vi "ConfigureLowRateAnalysis.vi"(8 "error in (no error)":errorcluster) -> (0 "error out":errorcluster, 2 "register trends":T1[](array[typedef]), 3 "analysis config":T3, 5 "all config found?":bool)   [LabVIEW 2017, in "McsaAnalysisLowRate.lvlib"]
uses:
  <vilib>/addons/InsightCM/Devices/Shared/Mcsa/McsaAnalysisLowRate/McsaAnalysisLowRate.lvlib
  <vilib>/addons/InsightCM/Utilities/GlobalConfiguration/GlobalConfiguration.lvlib
  <vilib>/addons/InsightCM/Utilities/DeviceModelHelpers/DeviceModelHelpers.lvlib
  <vilib>/addons/InsightCM/Utilities/Analysis/Shared/AnalysisHelper.lvlib
  <vilib>/addons/InsightCM/Devices/Shared/Mcsa/McsaVirtualChannel/McsaVirtualChannel.lvlib
  <vilib>/addons/InsightCM/Utilities/Analysis/MCSA/McsaAnalysisFunctions.lvlib
  <vilib>/addons/InsightCM/Utilities/Analysis/Shared/controls/AmplitudeScale.ctl
  <vilib>/addons/InsightCM/Utilities/Analysis/Shared/controls/Feature.ctl
  <vilib>/addons/InsightCM/Utilities/Analysis/MCSA/controls/McsaChannelPhasor.ctl
  <vilib>/addons/InsightCM/Devices/Shared/Mcsa/McsaAnalysisLowRate/controls/Group.ctl
  <vilib>/addons/InsightCM/Utilities/Analysis/MCSA/controls/WorkingCurrent.ctl
  <vilib>/addons/InsightCM/Devices/Shared/Mcsa/McsaAnalysisLowRate/controls/Config.ctl
  <vilib>/addons/InsightCM/Utilities/Analysis/MCSA/controls/McsaChannel.ctl
  <vilib>/addons/InsightCM/MessageBus/Base/controls/KeyValuePair.ctl
  <vilib>/addons/InsightCM/Utilities/Analysis/MCSA/controls/McsaMotor.ctl
  <vilib>/addons/InsightCM/Utilities/Analysis/MCSA/controls/TorqueLoadEfficiency.ctl
  <vilib>/addons/Electrical Power/Basic/Measurement/subVIs/basic_Power Value.ctl
  <vilib>/addons/Electrical Power/Basic/NI_EP_Basic.lvlib
  <vilib>/addons/InsightCM/Utilities/Analysis/MCSA/controls/MotorCalculationCache.ctl
  <vilib>/addons/InsightCM/Devices/Shared/Common/DataEventCreator/controls/Registry_Trend.ctl
  <vilib>/addons/InsightCM/Devices/Shared/Common/DataEventCreator/DataEventCreator.lvlib
  <vilib>/addons/InsightCM/Devices/Shared/Common/DataEventCreator/controls/RegisterTrendPoints.ctl
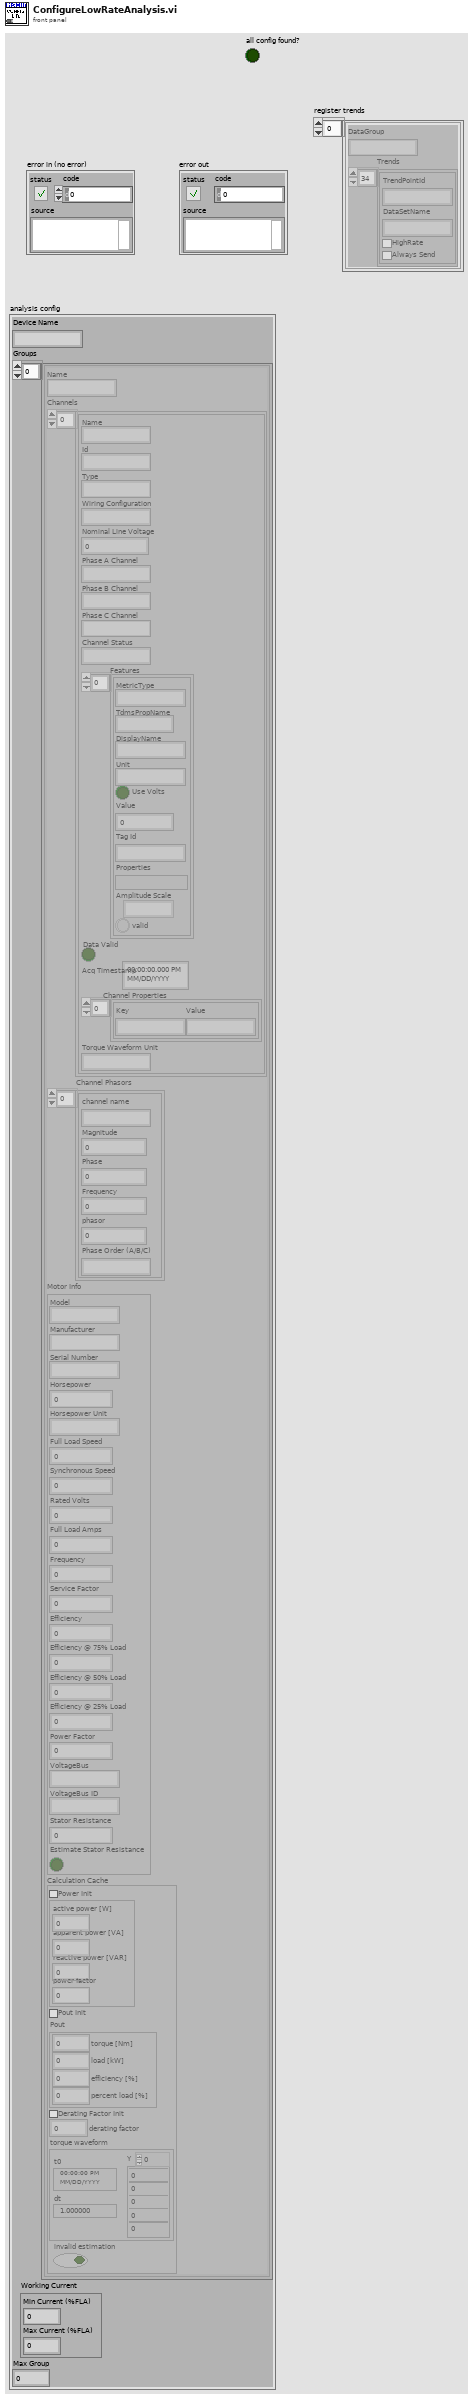
[diagram p1: front panel]
types:
  T1 = typedef "DataEventCreator.lvlib/RegisterTrendPoints.ctl" = cluster{"DataGroup":string, "Trends":T2[]}
  T2 = typedef "DataEventCreator.lvlib/Registry_Trend.ctl" = cluster{"TrendPointId":string, "DataSetName":string, "HighRate":bool, "Always Send":bool}
  T3 = typedef "McsaAnalysisLowRate.lvlib/Config.ctl" = cluster{"Device Name":string, "Groups":T4[], "Working Current":T14, "Max Group":i32}
  T4 = typedef "McsaAnalysisLowRate.lvlib/Group.ctl" = cluster{"Name":string, "Channels":T5[], "Channel Phasors":T9[], "Motor Info":T10, "Calculation Cache":T11}
  T5 = typedef "McsaAnalysisFunctions.lvlib/McsaChannel.ctl" = cluster{"Name":string, "Id":string, "Type":string, "Wiring Configuration":string, "Nominal Line Voltage":dbl, "Phase A Channel":string, "Phase B Channel":string, "Phase C Channel":string, "Channel Status":string, "Features":T6[], "Data Valid":bool, "Acq Timestamp":timestamp, "Channel Properties":T8[], "Torque Waveform Unit":string}
  T6 = typedef "AnalysisHelper.lvlib/Feature.ctl" = cluster{"MetricType":string, "TdmsPropName":string, "DisplayName":string, "Unit":string, "Use Volts":bool, "Value":dbl, "Tag Id":string, "Properties":variant, "Amplitude Scale":T7, "valid":bool}
  T7 = typedef "AnalysisHelper.lvlib/AmplitudeScale.ctl" = enum16{"rms", "peak", "pk-pk"}
  T8 = typedef "KeyValuePair.ctl" = cluster{"Key":string, "Value":string}
  T9 = typedef "McsaAnalysisFunctions.lvlib/McsaChannelPhasor.ctl" = cluster{"channel name":string, "Magnitude":dbl, "Phase":dbl, "Frequency":dbl, "phasor":cdb, "Phase Order (A/B/C)":string}
  T10 = typedef "McsaAnalysisFunctions.lvlib/McsaMotor.ctl" = cluster{"Model":string, "Manufacturer":string, "Serial Number":string, "Horsepower":dbl, "Horsepower Unit":string, "Full Load Speed":dbl, "Synchronous Speed":dbl, "Rated Volts":dbl, "Full Load Amps":dbl, "Frequency":dbl, "Service Factor":dbl, "Efficiency":dbl, "Efficiency @ 75% Load":dbl, "Efficiency @ 50% Load":dbl, "Efficiency @ 25% Load":dbl, "Power Factor":dbl, "VoltageBus":string, "VoltageBus ID":string, "Stator Resistance":dbl, "Estimate Stator Resistance":bool}
  T11 = typedef "McsaAnalysisFunctions.lvlib/MotorCalculationCache.ctl" = cluster{"Power Init":bool, "power value":T12, "Pout Init":bool, "Pout":T13, "Derating Factor Init":bool, "derating factor":sgl, "torque waveform":waveform(dbl), "invalid estimation":bool}
  T12 = typedef "NI_EP_Basic.lvlib/basic_Power Value.ctl" = cluster{"active power [W]":dbl, "apparent power [VA]":dbl, "reactive power [VAR]":dbl, "power factor":dbl}
  T13 = typedef "McsaAnalysisFunctions.lvlib/TorqueLoadEfficiency.ctl" = cluster{"torque [Nm]":dbl, "load [kW]":dbl, "efficiency [%]":dbl, "percent load [%]":dbl}
  T14 = typedef "McsaAnalysisFunctions.lvlib/WorkingCurrent.ctl" = cluster{"Min Current (%FLA)":dbl, "Max Current (%FLA)":dbl}
  T15 = typedef "R2_DeviceModel.ctl" = cluster{"Device":T16, "Channels":T23[], "Tags":T25[]}
  T16 = typedef "R2_Device.ctl" = cluster{"Id":string, "Name":string, "DeviceType":string, "HardwareName":string, "IpAddress":string, "HardwareInfo":T8[], "ApplicationType":string, "ApplicationVersion":string, "EquipmentIds":string[], "ConfigurationVersion":string, "State":T17, "Properties":T8[], "DataGroups":T18[], "BurstModeTrigger":T22}
  T17 = typedef "DeviceState.ctl" = cluster{"Disabled":bool}
  T18 = typedef "R2_DataGroup.ctl" = cluster{"Name":string, "OperatingStates":T19[], "Properties":T8[], "EquipmentIds":string[], "AssetNodeId":string}
  T19 = typedef "OperatingState.ctl" = cluster{"Name":string, "Properties":T8[], "Triggers":T20[]}
  T20 = typedef "Trigger.ctl" = cluster{"Type":string, "Expression":string, "Conditions":T21[]}
  T21 = typedef "Condition.ctl" = cluster{"Source":string, "Type":string, "Operator":string, "CompareTo":string, "DwellSeconds":dbl}
  T22 = typedef "BurstModeTrigger.ctl" = cluster{"Trigger":T20, "SampleRate":string, "AcquisitionLength":string}
  T23 = typedef "R2_Channel.ctl" = cluster{"Id":string, "DeviceId":string, "Name":string, "ChannelType":string, "HardwareKey":string, "HardwareChannel":string, "DataGroup":string, "Keywords":string[], "EquipmentIds":string[], "Properties":T8[], "Metrics":T24[], "AssetNodeId":string, "MeasType":string, "AssetName":string}
  T24 = typedef "Metric.ctl" = cluster{"Id":string, "Name":string, "Unit":string, "Properties":T8[], "MetricDefinitionInstanceId":string}
  T25 = typedef "Tag.ctl" = cluster{"Id":string, "Path":string, "Name":string, "Datatype":string, "Props":T8[], "Keywords":string[]}
  T26 = typedef "SectionKeyValues.ctl" = cluster{"Section":string, "KeyValues":T8[]}
  T27 = typedef "MetricDefinitionInstance.ctl" = cluster{"Id":string, "MetricType":string, "Name":string, "Properties":T8[], "HighRate":bool}
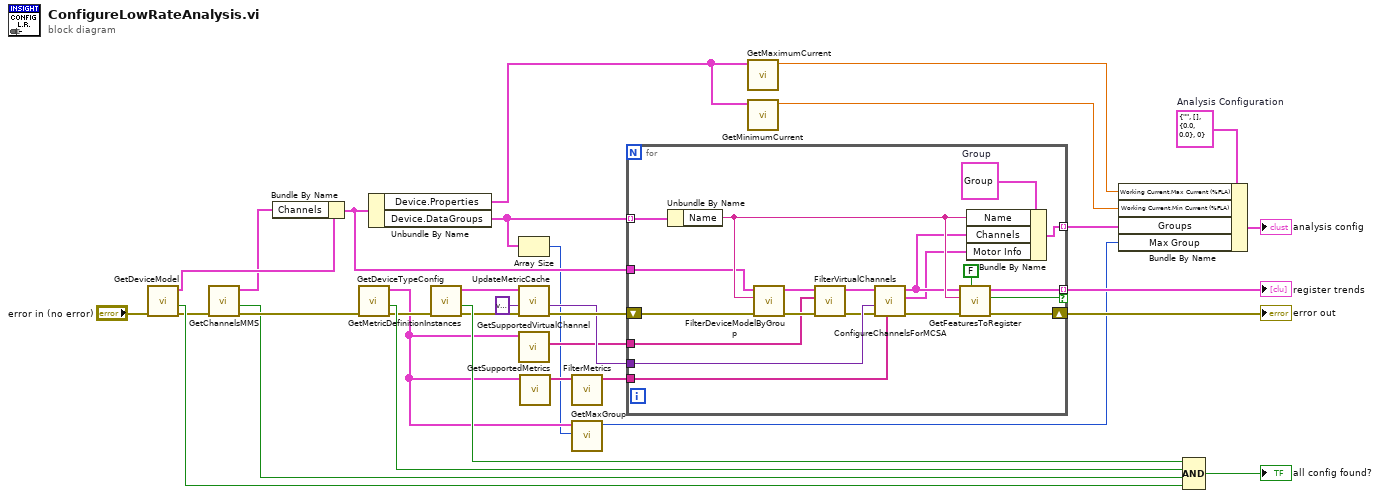
[diagram p0: block diagram]
diagram:
  w10 = T3 {"Device Name"="", "Groups"=[], "Working Current"={"Min Current (%FLA)"=0.0, "Max Current (%FLA)"=0.0}, "Max Group"=0}  # Analysis Configuration
  n1 = call <vilib>:"GetDeviceModel.vi"("error in (no error)"="error in (no error)") -> ("error out"=w13:errorcluster, "found"=w28:bool, "device model"=w15:T15)  [unwired: 8 in]
  n2 = call <vilib>:"GetChannelsMMS.vi"("error in (no error)"=w13) -> ("error out"=w12:errorcluster, "found"=w7:bool, "MMS Channels"=w11:T23[])  [unwired: 6 in, 2 out]
  n3 = Bundle By Name(cluster=w15, "Channels"=w11) -> (w14:T15)
  n4 = call <vilib>:"GetDeviceTypeConfig.vi"("error in (no error)"=w12) -> ("error out"=w18:errorcluster, "found"=w26:bool, "key values"=w4:T26[])  [unwired: 8 in]
  n5 = Unbundle By Name(w14) -> ("Device.Properties"=w5:T8[], "Device.DataGroups"=w3:T18[])
  n6 = call <vilib>:"GetMetricDefinitionInstances.vi"("error in (no error)"=w18) -> ("error out"=w24:errorcluster, "found"=w27:bool, "metrics"=w22:T27[])  [unwired: 8 in]
  n7 = Array Size(array=w3) -> (size(s)=w2:i32)
  n8 = call <vilib>:"UpdateMetricCache.vi"("error in (no error)"=w24, "Metrics"=variant, "MetricDefinitionInstances"=w22) -> ("error out"=w23:errorcluster, "Metrics out"=w21:variant)  [unwired: 7 in]
  n9 = call <vilib>:"GetSupportedVirtualChannel.vi"("key values"=w4) -> ("not supported virtual channels"=w17:string[])  [unwired: 9 in, 1 out]
  n10 = call <vilib>:"GetSupportedMetrics.vi"("key values"=w4) -> ("supported metrics"=w16:string[])  [unwired: 10 in]
  n11 = call <vilib>:"FilterMetrics.vi"("supported metrics"=w16) -> ("low-rate supported metrics"=w6:string[])  [unwired: 9 in, 1 out]
  n12 = call <vilib>:"GetMaxGroup.vi"("total groups"=w2, "key values"=w4) -> ("Max Group"=w1:i32)  [unwired: 9 in]
  n13 = for {
    tunnel: w21 -> [w52]
    tunnel: w14 -> [w38]
    shift-right: [w49] -> w32
    shift-left: w23 -> [w50]
    tunnel: [w51] -> w19 mode=indexing
    tunnel: w3 -> [w36] mode=indexing
    tunnel: [w48] -> w31 mode=indexing if=w47
    tunnel: w6 -> [w45]
    tunnel: w17 -> [w39]
    w35 = T4 {"Name"="", "Channels"=[], "Channel Phasors"=[], "Motor Info"={"Model"="", "Manufacturer"="", "Serial Number"="", "Horsepower"=0.0, "Horsepower Unit"="", "Full Load Speed"=0.0, "Synchronous Speed"=0.0, "Rated Volts"=0.0, "Full Load Amps"=0.0, "Frequency"=0.0, "Service Factor"=0.0, "Efficiency"=0.0, "Efficiency @ 75% Load"=0.0, "Efficiency @ 50% Load"=0.0, "Efficiency @ 25% Load"=0.0, "Power Factor"=0.0, "VoltageBus"="", "VoltageBus ID"="", "Stator Resistance"=0.0, "Estimate Stator Resistance"=FALSE}, "Calculation Cache"={"Power Init"=FALSE, "power value"={"active power [W]"=0.0, "apparent power [VA]"=0.0, "reactive power [VAR]"=0.0, "power factor"=0.0}, "Pout Init"=FALSE, "Pout"={"torque [Nm]"=0.0, "load [kW]"=0.0, "efficiency [%]"=0.0, "percent load [%]"=0.0}, "Derating Factor Init"=FALSE, "derating factor"=0.0, "torque waveform"={"t0"=timestamp(0 s since 1904-01-01), "dt"=1.0, "Y"=[]}, "invalid estimation"=FALSE}}  # Group
    n14 = Unbundle By Name(w36) -> ("Name"=w46:string)
    n15 = call <vilib>:"FilterDeviceModelByGroup.vi"("error in (no error)"=w50, "group"=w46, "device model"=w38) -> ("error out"=w40:errorcluster, "device model (channels filtered by group)"=w42:T15)  [unwired: 7 in]
    n16 = call <vilib>:"FilterVirtualChannels.vi"("error in (no error)"=w40, "not supported virtual channels"=w39, "device model"=w42) -> ("error out"=w41:errorcluster, "device model (unsupported virtual channels filtered out)"=w43:T15)  [unwired: 7 in]
    n17 = call <vilib>:"ConfigureChannelsForMCSA.vi"("Supported Metrics"=w45, "error in (no error)"=w41, "metric cache"=w52, "device"=w43) -> ("error out"=w44:errorcluster, "Motor Info Out"=w33:T10, "channels"=w34:T5[])  [unwired: 5 in]
    n18 = call <vilib>:"GetFeaturesToRegister.vi"("high rate"=FALSE, "error in (no error)"=w44, "group"=w46, "channels"=w34) -> ("error out"=w49:errorcluster, "atleast one"=w47:bool, "register trend"=w48:T1)  [unwired: 5 in]
    n19 = Bundle By Name(cluster=w35, "Name"=w46, "Channels"=w34, "Motor Info"=w33) -> (w51:T4)
  }
  "error out" <- w32
  "register trends" <- w31
  n20 = call <vilib>:"GetMaximumCurrent.vi"("Properties"=w5) -> ("Maximum Current (%FLA)"=w8:dbl)  [unwired: 10 in]
  n21 = call <vilib>:"GetMinimumCurrent.vi"("Properties"=w5) -> ("Minimum Current (%FLA)"=w9:dbl)  [unwired: 10 in]
  n22 = Bundle By Name(cluster=w10, "Working Current.Max Current (%FLA)"=w8, "Working Current.Min Current (%FLA)"=w9, "Groups"=w19, "Max Group"=w1) -> (→"analysis config":T3)
  n23 = Compound Arithmetic op=AND(w27, w26, w7, w28) -> (→"all config found?":bool)
